vi "TestSyncTurn.vi"() -> ()   [LabVIEW 2017]
uses:
  Projekt-RubikLibrary/ServoCCWControl.ctl
  Projekt-RubikLibrary/ServoEnumControl.ctl
  Projekt-RubikLibrary/ServoAbsAngleControl.ctl
  Projekt-RubikLibrary/RubikLibraryRT.lvlib
  Projekt-RubikLibrary/RubikLibrary.lvlib
panel:
  in  "Turn to (in)":T1
  in  "stop":bool
  # "Test Asynchronous Behaviour of Grip Servos\n\n\"Asynchronous\" means that VI(software) does not\nwait (default 500ms). Actually you will observe\nsynchronous behaviour: all three grips will move\nsynchronously. But the VI does not wait for completion \nof grip.\n\n\"NoWait==T\" means grips execute in parallel\n\"NoWait==F\" shows one grip after the other."
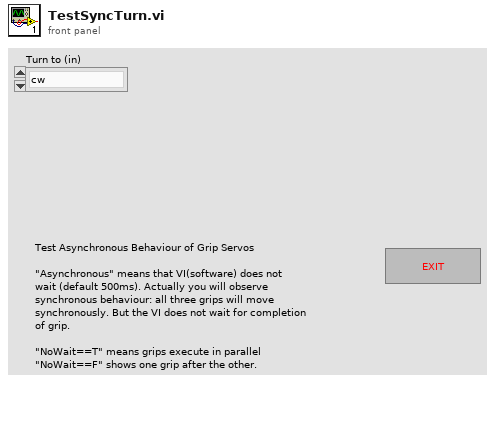
[diagram p1: front panel]
types:
  T1 = typedef "RubikLibrary.lvlib/ServoCCWControl.ctl" = enum16{"cw", "ccw"}
  T2 = typedef "RubikLibrary.lvlib/ServoAbsAngleControl.ctl" = enum16{"+90°", "0°", "-90°"}
  T3 = typedef "RubikLibrary.lvlib/ServoEnumControl.ctl" = enum16{"Left Servo", "Front Servo", "Right Servo"}
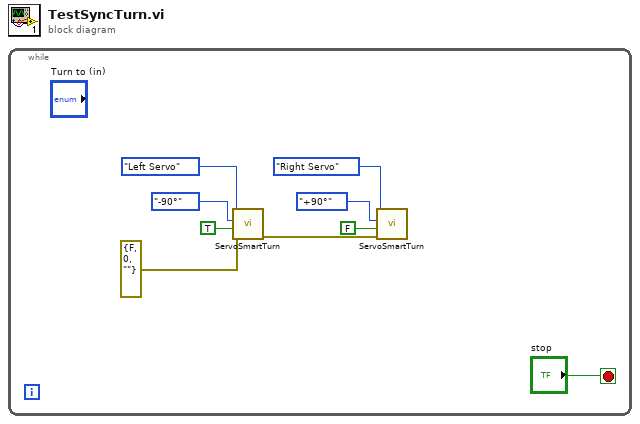
[diagram p0: block diagram]
diagram:
  n1 = while {
    stop <- "stop" stop-if-true
    n2 = call "ServoSmartTurn.vi"("error in"=errorcluster {"status"=FALSE, "code"=0, "source"=""}, "NoWait"=TRUE, "Turn to (in)"=ServoAbsAngleControl."-90°", "Servo"=ServoEnumControl."Left Servo") -> ("error out"=w7:errorcluster)  [unwired: 6 in, 1 out]
    n3 = call "ServoSmartTurn.vi"("error in"=w7, "NoWait"=FALSE, "Turn to (in)"=ServoAbsAngleControl."+90°", "Servo"=ServoEnumControl."Right Servo") -> ()  [unwired: 6 in, 2 out]
  }
